vi "PD SYNC DAQ.vi"(3 "Custom Range (0 V)":dbl=10.0 format="%#_6p", 6 "Addition info":string, 7 "X-pixel size(um).":dbl, 8 "VISA resource name":refnum<visa-resource-name>="GPIB::16", 9 "samples per channel":i32=100, 10 "Trigger events":i32, 11 "Counter(s)":tag="Dev1/ctr4") -> (0 "Intensity Graph":dbl[][](graph), 1 "Data":dbl[](array[numeric]))   [LabVIEW 2011]
doc: "I. Description:\nThis example demonstrates how to generate a continuous digital pulse train from a Counter Output Channel. The Frequency, Duty Cycle, and Idle State are all configurable. \n\nThis example shows how to configure the pulse in terms of Frequency/Duty Cycle, but can easily be modified to generate a pulse in terms of Time or Ticks.\n\nII. Instructions for Running:\n1. Select the Physical Channel which corresponds to the counter you want to output your signal to on the DAQ device.\n2. Enter the Frequency and Duty Cycle to define the pulse parameters. You can also change the Idle State to determine the beginning and end states of the output. If the Idle State is High, the generation will use inverted logic. Additionally, you can set the Initial Delay (in seconds) which will delay the beginning of the pulse train from the start call; this is currently wired to 0.0 on the diagram. \nNote: Use the Measure Period example to verify you are outputting the pulse train on the DAQ device.\n\nIII. Block Diagram Steps:\n1. Create a Counter Output channel to produce a Pulse in terms of Frequency. If the Idle State of the pulse is set to low, the state of the line will begin low and remain low after the generation is stopped.\n2. Use the DAQmx Timing VI (Implicit) to configure the duration of the pulse generation.\n3. Call the Start VI to arm the counter and begin the pulse train generation.\n4. Loop continuously until the user presses the Stop button. Check for errors every 100 ms using the Is Task Done? VI\n5. Call the Clear Task VI to clear the Task.\n\nIV. I/O Connections Overview:\nThe counter will output the pulse train on the output terminal of the counter specified in the Physical Channel I/O control. \n\nIn this example the output will be sent to the default output terminal on ctr0.\n\nFor more information on the default counter input and output terminals for your device, open the NI-DAQmx Help, and refer to Counter Signal Connections found under the Device Considerations book in the table of contents."
uses:
  <vilib>/Utility/error.llb/DialogType.ctl
  <vilib>/Utility/file.llb/Write To Spreadsheet File (DBL).vi
  <vilib>/DAQmx/create/channels.llb/DAQmx Create Channel (CO-Pulse Generation-Frequency).vi
  <vilib>/DAQmx/configure/timing.llb/DAQmx Timing (Implicit).vi
  <userlib>/Keithley 2000 Series (3.0.0) LV8.0+/Public/Configure/Configure DC Volts.vi
  <userlib>/Keithley 2000 Series (3.0.0) LV8.0+/Keithley 2000.lvlib
  C:/Program Files (x86)/National Instruments/LabVIEW 2011/resource/objmgr/daqmx.rc
panel:
  in  "Saving Path":string="D:\\顯微鏡\\Data\\"
  out "X step":string
  in  "Detector type":string="PD_"
  out "Nth loop":i32
  # "PD"
  # "DAQ setting"
  # "Channel Parameters"
  # "These parameters are set\nbefore running the example."
  # "Mutimeter setting"
  # "存檔路徑"
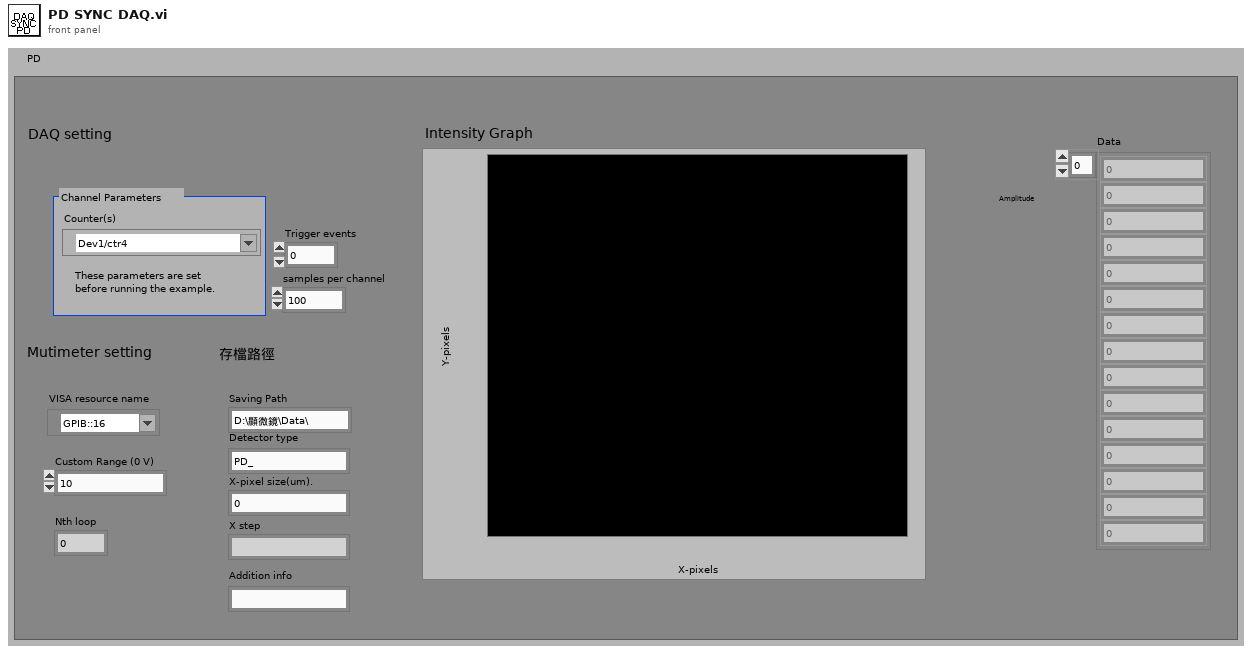
[diagram p1: front panel]
types:
  T1 = typedef "DialogType.ctl" = u16
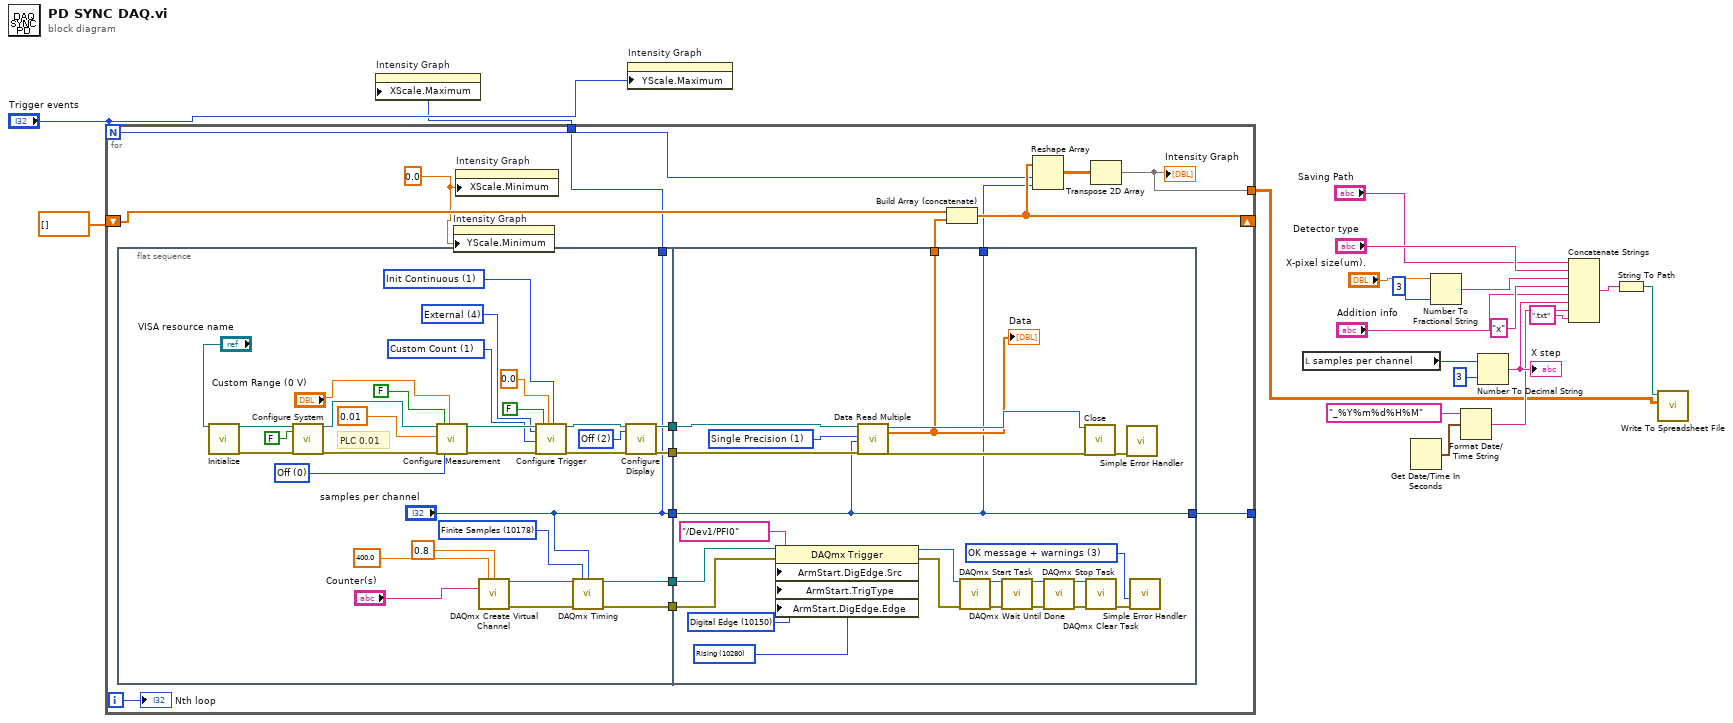
[diagram p0: block diagram]
diagram:
  n1 = for {
    N: "Trigger events" -> [w25]
    shift-right: [w27] -> _
    shift-left: dbl[] [] -> [w30]
    tunnel: [w29] -> _
    tunnel: [w23] -> w4
    tunnel: [w21] -> w2
    i -> [w28]
    w22 = 0.0 ("X Scale.Range:Minimum")
    n2 = flat-sequence {
      tunnel: [w47] -> w36
      tunnel: [w46] -> w35
      tunnel: [w41] -> w34
      tunnel: [w40] -> w33
      tunnel: ["samples per channel"] -> w32
      tunnel: ["samples per channel"] -> w21
      tunnel: w36 -> [w81]
      tunnel: w35 -> [w82]
      tunnel: w34 -> [w73]
      tunnel: w33 -> [w72]
      tunnel: w32 -> [w68]
      tunnel: [w76] -> w31
      tunnel: [w68] -> w29
      tunnel: [w68] -> w26
      frame #0 {
        w39 = 10178 items=["Finite Samples"=10178, "Continuous Samples"=10123] ("sample mode")
        w48 = u16 1 items=["Infinite", "Custom Count"] ("Count Mode (0: Infinite)")
        w50 = u16 2 items=["Normal", "Text", "Off"] ("Display (0: Normal)")
        w51 = i16 1 items=["Don't Init"=-1, "Init Single"=0, "Init Continuous"=1] ("Init (1: Init Continuous)")
        w63 = u16 0 items=["Off", "Moving Filter", "Repeating Filter"] ("Digital Filter (0: Off)")
        w65 = u16 4 items=["Immediate", "Timer", "Manual", "Bus", "External"] ("Source (0: Immediate)")
        # "PLC 0.01"
        n3 = call <userlib>:"Initialize.vi"("VISA resource name"="VISA resource name") -> ("VISA resource name out"=w59:refnum<visa-resource-name>, "error out"=w62:errorcluster)  [unwired: 17 in]
        n4 = call <userlib>:"Configure System.vi"("VISA resource name"=w59, "Autozero Enabled? (T: On)"=FALSE, "error in (no error)"=w62) -> ("VISA resource name out"=w60:refnum<visa-resource-name>, "error out"=w61:errorcluster)  [unwired: 15 in]
        n5 = call-poly <userlib>:"Configure Measurement.vi"("VISA resource name"=w60, "Power Line Cycles (1.00)"=0.01, "error in (no error)"=w61, "Auto Range? (T: Auto)"=FALSE, "Digital Filter (0: Off)"=w63, "Custom Range (0 V)"="Custom Range (0 V)") -> ("VISA resource name out"=w66:refnum<visa-resource-name>, "error out"=w64:errorcluster)  [unwired: 12 in]
        n6 = call-poly <vilib>:"DAQmx Create Virtual Channel.vi"("frequency"=400.0, "duty cycle"=0.8, "counter"="Counter(s)") -> ("task out"=w43:refnum<k21>, "error out"=w42:errorcluster)  [unwired: 11 in]
        n7 = call <userlib>:"Configure Trigger.vi"("VISA resource name"=w66, "Source (0: Immediate)"=w65, "Count Mode (0: Infinite)"=w48, "error in (no error)"=w64, "Auto Delay? (F: Custom)"=FALSE, "Delay (0 s)"=0.0, "Init (1: Init Continuous)"=w51) -> ("VISA resource name out"=w52:refnum<visa-resource-name>, "error out"=w53:errorcluster)  [unwired: 11 in]
        n8 = call-poly <vilib>:"DAQmx Timing.vi"("task/channels in"=w43, "sample mode"=w39, "samples per channel"="samples per channel", "error in"=w42) -> ("task out"=w41:refnum<k21>, "error out"=w40:errorcluster)  [unwired: 10 in]
        n9 = call <userlib>:"Configure Display.vi"("VISA resource name"=w52, "Display (0: Normal)"=w50, "error in (no error)"=w53) -> ("VISA resource name out"=w47:refnum<visa-resource-name>, "error out"=w46:errorcluster)  [unwired: 15 in]
      }
      frame #1 {
        w69 = 10280 items=["Rising"=10280, "Falling"=10171] ("ArmStart.DigEdge.Edge")
        w70 = 10150 items=["Digital Edge"=10150, "None"=10230] ("ArmStart.TrigType")
        w86 = u16 1 items=["ASCII", "Single Precision", "Double Precision"] ("Format (0: ASCII)")
        w89 = T1 3 items=["no dialog", "OK message", "continue or stop message", "OK message + warnings", "continue/stop + warnings"] ("type of dialog (OK msg:1)")
        n10 = property class="DAQmx Trigger"(reference=w73, error in=w72, "ArmStart.DigEdge.Src"=tag "/Dev1/PFI0", "ArmStart.TrigType"=w70, "ArmStart.DigEdge.Edge"=w69) -> (reference out=w75:refnum<k21>, error out=w74:errorcluster)
        n11 = call <userlib>:"Data Read Multiple.vi"("VISA resource name"=w81, "Format (0: ASCII)"=w86, "Number of Readings (100)"=w68, "error in (no error)"=w82) -> ("VISA resource name out"=w85:refnum<visa-resource-name>, "Data"=w76:dbl[], "error out"=w84:errorcluster)  [unwired: 11 in, 2 out]
        "Data" <- w76
        n12 = call <vilib>:"DAQmx Start Task.vi"("task/channels in"=w75, "error in"=w74) -> ("task out"=w80:refnum<k21>, "error out"=w79:errorcluster)  [unwired: 12 in]
        n13 = call <vilib>:"DAQmx Wait Until Done.vi"("task/channels in"=w80, "error in"=w79) -> ("task out"=w77:refnum<k21>, "error out"=w78:errorcluster)  [unwired: 12 in]
        n14 = call <vilib>:"DAQmx Stop Task.vi"("task/channels in"=w77, "error in"=w78) -> ("task out"=w87:refnum<k21>, "error out"=w88:errorcluster)  [unwired: 12 in]
        n15 = call <userlib>:"Close.vi"("VISA resource name"=w85, "error in (no error)"=w84) -> ("error out"=w83:errorcluster)  [unwired: 17 in]
        n16 = call <vilib>:"DAQmx Clear Task.vi"("task in"=w87, "error in"=w88) -> ("error out"=w90:errorcluster)  [unwired: 13 in]
        n17 = call <vilib>:"Simple Error Handler.vi"("error in (no error)"=w83) -> ()  [unwired: 4 in, 5 out]
        n18 = call <vilib>:"Simple Error Handler.vi"("type of dialog (OK msg:1)"=w89, "error in (no error)"=w90) -> ()  [unwired: 3 in, 5 out]
      }
    }
    n19 = property on="Intensity Graph" class="IntGraph (strict)"("YScale.Minimum"=w22) -> ()  [unwired: 2 in, 2 out]
    n20 = property on="Intensity Graph" class="IntGraph (strict)"("XScale.Minimum"=w22) -> ()  [unwired: 2 in, 2 out]
    n21 = Build Array (concatenate)(w30, w31) -> (w27:dbl[])
    n22 = Reshape Array(w27, w25, w26) -> (w24:dbl[][])
    n23 = Transpose 2D Array(2D array=w24) -> (transposed array=w23:dbl[][])
    "Intensity Graph" <- w23
    "Nth loop" <- w28
  }
  n24 = property on="Intensity Graph" class="IntGraph (strict)"("XScale.Maximum"=w2) -> ()  [unwired: 2 in, 2 out]
  n25 = property on="Intensity Graph" class="IntGraph (strict)"("YScale.Maximum"="Trigger events") -> ()  [unwired: 2 in, 2 out]
  n26 = local read "samples per channel"() -> (w5:i32)
  n27 = Get Date/Time In Seconds() -> (seconds since 1Jan1904=w14:timestamp)
  n28 = Number To Fractional String(number="X-pixel size(um).", precision (6)=i16 3 ("width (-)")) -> (F-format string=w13:string)  [unwired: 2 in]
  n29 = Format Date/Time String(time format string (%c)="_%Y%m%d%H%M", seconds (now)=w14) -> (date/time string=w17:string)  [unwired: 1 in]
  n30 = Number To Decimal String(number=w5, width (-)=i16 3) -> (decimal integer string=w18:string)
  "X step" <- w18
  n31 = Concatenate Strings("Saving Path", "Detector type", w13, "x", "Addition info", w18, w17, ".txt" ("string")) -> (w10:string)
  n32 = String To Path(string=w10) -> (path=w11:path)
  n33 = call-poly <vilib>:"Write To Spreadsheet File.vi"("2D data"=w4, "file path (dialog if empty)"=w11) -> ()  [unwired: 6 in, 1 out]
